vi "状态读取.vi"   [LabVIEW 2020]
uses:
  Global_Variable/Global.vi
types:
  T1 = cluster{"空载角度":sgl, "空载速度":sgl, "工装移载位移":sgl, "输入编码位移":sgl, "输入扭矩":sgl, "123":sgl, "拉压力":sgl, "吸收电流":sgl}
  T2 = cluster{"左工位驱动伺服位移":sgl, "右工位驱动伺服位移":sgl, "横向伺服位移":sgl, "左加载伺服位移":sgl, "右加载伺服位移":sgl}
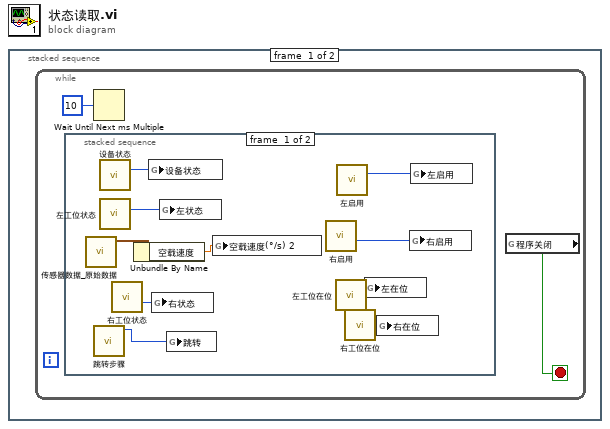
[diagram p0: block diagram]
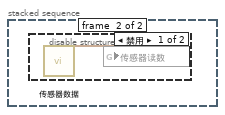
[diagram p2: hidden frame]
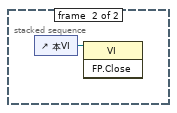
[diagram p4: hidden frame]
diagram:
  n1 = stacked-sequence {
    frame #0 {
      n2 = while {
        stop <- w1 stop-if-true
        n3 = stacked-sequence {
          frame #0 {
            n4 = call "传感器数据_原始数据.vi"() -> ("传感器读数"=w4:T1)  [unwired: 11 in]
            n5 = call "跳转步骤.vi"() -> ("Status_Read"=w9:i16)  [unwired: 11 in]
            n6 = call "设备状态.vi"() -> ("Status_Read"=w12:i16)  [unwired: 11 in]
            n7 = call "左工位状态.vi"() -> ("Status_Read"=w11:i16)  [unwired: 11 in]
            n8 = call "右工位状态.vi"() -> ("Status_Read"=w10:i16)  [unwired: 11 in]
            n9 = Unbundle By Name(w4) -> ("空载速度"=w3:sgl)
            n10 = global write "Global.vi" "设备状态"(w12) -> ()
            n11 = global write "Global.vi" "右状态"(w10) -> ()
            n12 = global write "Global.vi" "左状态"(w11) -> ()
            n13 = global write "Global.vi" "跳转"(w9) -> ()
            n14 = global write "Global.vi" "空载速度(°/s) 2"(w3) -> ()
            n15 = call "右启用.vi"() -> ("Status_Read"=w7:i16)  [unwired: 11 in]
            n16 = call "左工位在位.vi"() -> ("Status_Read"=w5:i16)  [unwired: 11 in]
            n17 = call "左启用.vi"() -> ("Status_Read"=w8:i16)  [unwired: 11 in]
            n18 = call "右工位在位.vi"() -> ("Status_Read"=w6:i16)  [unwired: 11 in]
            n19 = global write "Global.vi" "左在位"(w5) -> ()
            n20 = global write "Global.vi" "右在位"(w6) -> ()
            n21 = global write "Global.vi" "右启用"(w7) -> ()
            n22 = global write "Global.vi" "左启用"(w8) -> ()
          }
          frame #1 {
            n23 = disable-structure shown="禁用" {
              frame Disabled {
                n24 = call "传感器数据.vi"() -> ("传感器读数"=w13:T2)  [unwired: 11 in]
                n25 = global write "Global.vi" "传感器读数"(w13) -> ()
              }
              frame Enabled {
              }
            }
          }
        }
        n26 = Wait Until Next ms Multiple(millisecond multiple=u32 10 ("毫秒倍数")) -> ()  [unwired: 1 out]
        n27 = global read "Global.vi" "程序关闭"() -> (w1:bool)
      }
    }
    frame #1 {
      n28 = control-ref of="本VI"() -> (w14:refnum<vi>)
      n29 = invoke class="VI" method="FP.Close"(reference=w14) -> ()  [unwired: 2 in, 3 out]
    }
  }
